vi "Outlet Convert Temp to Volt.vi"(1 "Outlet Temperature":dbl) -> (0 "Outlet Voltage":dbl)   [LabVIEW 2014]
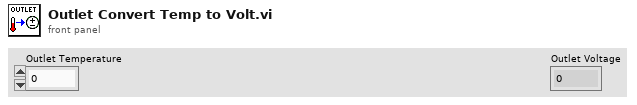
[diagram p1: front panel]
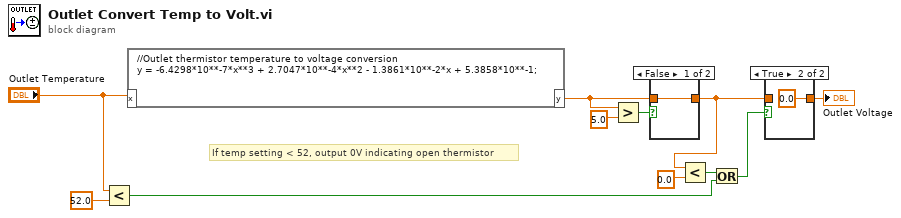
[diagram p0: block diagram]
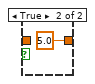
[diagram p3: hidden frame]
diagram:
  # "If temp setting < 52, output 0V indicating open thermistor"
  n1 = Less?(x="Outlet Temperature", y=52.0) -> (x < y?=w1:bool)
  n2 = formula code="//Outlet thermistor temperature to voltage conversion\ny = -6.4298*10**-7*x**3 + 2.7047*10**-4*x**2 - 1.3861*10**-2*x + 5.3858*10**-1;"("x"="Outlet Temperature") -> ("y"=w10:dbl)
  n3 = Greater?(x=w10, y=5.0) -> (0:w8:bool)
  n4 = case shown="False" w8 {
    tunnel: [w12 5.0 ("y")] -> w6
    tunnel: w10 -> [w12 _]
    frame False {
    }
    frame True {
    }
  }
  n5 = Less?(x=w6, y=0.0) -> (x < y?=w5:bool)
  n6 = Or(x=w5, y=w1) -> (x .or. y?=w4:bool)
  n7 = case shown="True" w4 {
    tunnel: [w14 0.0 ("y")] -> w7
    tunnel: w6 -> [w14 _]
    frame False {
    }
    frame True {
    }
  }
  "Outlet Voltage" <- w7
